vi "Drive Train Temps.vi"(8 "error in (no error)":errorcluster, 10 "Force Throttle?":bool, 11 "TalonSRX in":refnum<class "TalonSRX.lvclass">) -> (0 "error out":errorcluster, 2 "Drive Train Temperatures":T1={"Left Lead Temperature (C)"=nan, "Right Lead Temperature (C)"=nan, "Left Follows Temperatures (C)"=[], "Right Follows Temperatures (C)"=[]}, 3 "TalonSRX out":refnum<class "TalonSRX.lvclass">)   [LabVIEW 2019, in "Drive.lvlib" / "TalonSRX.lvclass"]
uses:
  TalonSRX.lvclass
  Controls/Drive Train Temperatures.ctl
  CTRE Drive.lvclass
  Tank Drive.lvclass
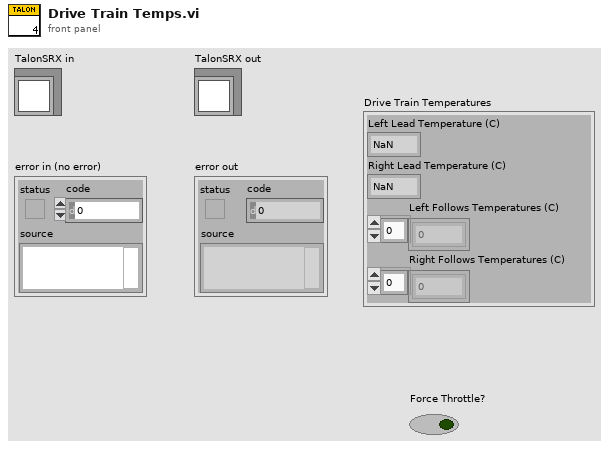
[diagram p1: front panel]
types:
  T1 = typedef "Drive.lvlib/Tank Drive.lvclass/Drive Train Temperatures.ctl" = cluster{"Left Lead Temperature (C)":dbl, "Right Lead Temperature (C)":dbl, "Left Follows Temperatures (C)":dbl[], "Right Follows Temperatures (C)":dbl[]}
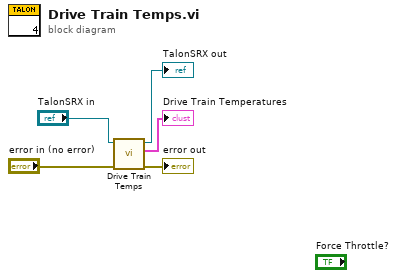
[diagram p0: block diagram]
diagram:
  n1 = call-parent "Drive Train Temps.vi"("error in (no error)"="error in (no error)", "Tank Drive in"="TalonSRX in") -> ("error out"=→"error out":errorcluster, "Drive Train Temperatures"=→"Drive Train Temperatures":T1, "Tank Drive out"=→"TalonSRX out":refnum<class "TalonSRX.lvclass">)  [unwired: 7 in]
